vi "Client Read.vi"(7 "force configure? (F)":bool, 8 "error in":errorcluster, 11 "connection ID in":T1) -> (0 "error out":errorcluster, 3 "connection ID out":T1)   [LabVIEW 2010, in "NI_CCC.lvlib"]
doc: "Requests the latest values of the read tag list from the CCC server, and applies the values to the local CVT."
uses:
  NI_CCC.lvlib
  Connection ID.ctl
  <vilib>/NI/STM/TCP/TCP Connection Info.ctl
  <vilib>/NI/STM/SubVIs/MetaDataElement.ctl
  Tag Configuration.ctl
  <vilib>/NI/Current Value Table/Type Defs/Data Types.ctl
  Tag Direction.ctl
  <vilib>/NI/STM/TCP/TCP Read Options.ctl
  <vilib>/NI/STM/TCP/TCP Write Options.ctl
  <vilib>/NI/Current Value Table/Type Defs/Group Data.ctl
  <vilib>/NI/Current Value Table/Write grouped data to tags.vi
  Read Error.vi
  Initialize Address_Index Lists.vi
  <vilib>/NI/Current Value Table/Write Index Set.vi
  <vilib>/NI/Current Value Table/DataTypes/Double_Write Index Set.vi
  <vilib>/NI/Current Value Table/DataTypes/Array of String_Write Index Set.vi
  <vilib>/NI/Current Value Table/DataTypes/Array of Boolean_Write Index Set.vi
  <vilib>/NI/Current Value Table/DataTypes/Array of Single_Write Index Set.vi
  <vilib>/NI/Current Value Table/DataTypes/Array of Double_Write Index Set.vi
  <vilib>/NI/Current Value Table/DataTypes/Array of I8_Write Index Set.vi
  <vilib>/NI/Current Value Table/DataTypes/Array of I16_Write Index Set.vi
  <vilib>/NI/Current Value Table/DataTypes/Array of I32_Write Index Set.vi
  <vilib>/NI/Current Value Table/DataTypes/Array of I64_Write Index Set.vi
  <vilib>/NI/Current Value Table/DataTypes/Array of U64_Write Index Set.vi
  <vilib>/NI/Current Value Table/DataTypes/Array of U32_Write Index Set.vi
  <vilib>/NI/Current Value Table/DataTypes/Array of U16_Write Index Set.vi
  <vilib>/NI/Current Value Table/DataTypes/Array of U8_Write Index Set.vi
  <vilib>/NI/Current Value Table/DataTypes/Boolean_Write Index Set.vi
  <vilib>/NI/Current Value Table/DataTypes/String_Write Index Set.vi
  <vilib>/NI/Current Value Table/DataTypes/U8_Write Index Set.vi
  <vilib>/NI/Current Value Table/DataTypes/U16_Write Index Set.vi
  <vilib>/NI/Current Value Table/DataTypes/U32_Write Index Set.vi
  <vilib>/NI/Current Value Table/DataTypes/U64_Write Index Set.vi
  <vilib>/NI/Current Value Table/DataTypes/I8_Write Index Set.vi
  <vilib>/NI/Current Value Table/DataTypes/I16_Write Index Set.vi
  <vilib>/NI/Current Value Table/DataTypes/I32_Write Index Set.vi
  <vilib>/NI/Current Value Table/DataTypes/I64_Write Index Set.vi
  <vilib>/NI/Current Value Table/DataTypes/Single_Write Index Set.vi
  <vilib>/NI/Current Value Table/Get Index and Type.vi
  <vilib>/NI/Current Value Table/Group Tags.vi
  <vilib>/Utility/error.llb/Error Cluster From Error Code.vi
  FG Client Configurations.vi
  <vilib>/NI/Current Value Table/FGVs/Tag Memory.vi
  <vilib>/NI/Current Value Table/FGVs/Group Memory.vi
  <vilib>/NI/Current Value Table/Form Single Group.vi
  <vilib>/NI/Current Value Table/Memory Block.vi
  <vilib>/NI/Current Value Table/DataTypes/Double_Memory Block.vi
  <vilib>/NI/Current Value Table/DataTypes/Array of String_Memory Block.vi
  <vilib>/NI/Current Value Table/DataTypes/Array of Boolean_Memory Block.vi
  <vilib>/NI/Current Value Table/DataTypes/Array of Single_Memory Block.vi
  <vilib>/NI/Current Value Table/DataTypes/Array of Double_Memory Block.vi
  <vilib>/NI/Current Value Table/DataTypes/Array of I8_Memory Block.vi
  <vilib>/NI/Current Value Table/DataTypes/Array of I16_Memory Block.vi
  <vilib>/NI/Current Value Table/DataTypes/Array of I32_Memory Block.vi
  <vilib>/NI/Current Value Table/DataTypes/Array of I64_Memory Block.vi
  <vilib>/NI/Current Value Table/DataTypes/Array of U64_Memory Block.vi
  <vilib>/NI/Current Value Table/DataTypes/Array of U32_Memory Block.vi
  <vilib>/NI/Current Value Table/DataTypes/Array of U16_Memory Block.vi
  <vilib>/NI/Current Value Table/DataTypes/Array of U8_Memory Block.vi
  <vilib>/NI/Current Value Table/DataTypes/Boolean_Memory Block.vi
  <vilib>/NI/Current Value Table/DataTypes/String_Memory Block.vi
  <vilib>/NI/Current Value Table/DataTypes/U8_Memory Block.vi
  <vilib>/NI/Current Value Table/DataTypes/U16_Memory Block.vi
  <vilib>/NI/Current Value Table/DataTypes/U32_Memory Block.vi
  <vilib>/NI/Current Value Table/DataTypes/U64_Memory Block.vi
  <vilib>/NI/Current Value Table/DataTypes/I8_Memory Block.vi
  <vilib>/NI/Current Value Table/DataTypes/I16_Memory Block.vi
  <vilib>/NI/Current Value Table/DataTypes/I32_Memory Block.vi
  <vilib>/NI/Current Value Table/DataTypes/I64_Memory Block.vi
  <vilib>/NI/Current Value Table/DataTypes/Single_Memory Block.vi
  <vilib>/NI/STM/NI STM.lvlib
  <vilib>/NI/Current Value Table/Current Value Table.lvlib
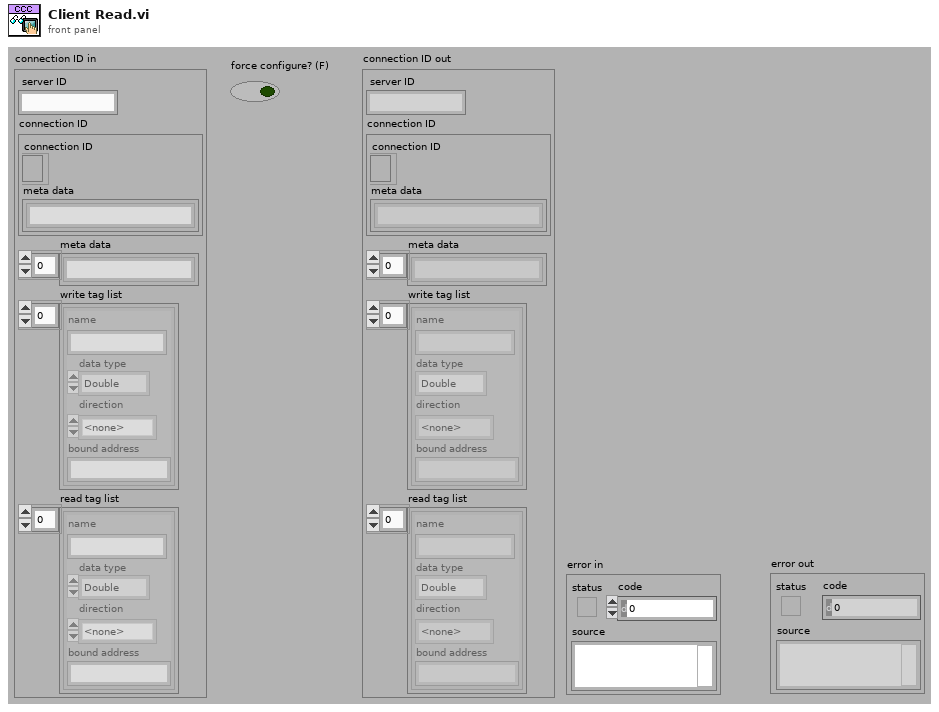
[diagram p1: front panel]
types:
  T1 = typedef "NI_CCC.lvlib/Connection ID.ctl" = cluster{"server ID":string, "connection ID":T2, "meta data":T3[], "write tag list":T4[], "read tag list":T4[]}
  T2 = typedef "NI STM.lvlib/TCP Connection Info.ctl" = cluster{"connection ID":refnum<k5>, "meta data":T3[]}
  T3 = typedef "NI STM.lvlib/MetaDataElement.ctl" = string
  T4 = typedef "NI_CCC.lvlib/Tag Configuration.ctl" = cluster{"name":string, "data type":T5, "direction":T6, "bound address":string}
  T5 = typedef "Current Value Table.lvlib/Data Types.ctl" = enum16{"Double", "Single", "I64", "I32", "I16", "I8", "U64", "U32", "U16", "U8", "String", "Boolean", "Array of U8", "Array of U16", "Array of U32", "Array of U64", "Array of I64", "Array of I32", "Array of I16", "Array of I8", "Array of Double", "Array of Single", "Array of Boolean", "Array of String"}
  T6 = typedef "NI_CCC.lvlib/Tag Direction.ctl" = enum32{"<none>", "Read", "Write"}
  T7 = typedef "NI STM.lvlib/TCP Read Options.ctl" = cluster{"ignore timeout error":bool, "timeout ms (1000)":i32}
  T8 = typedef "NI STM.lvlib/TCP Write Options.ctl" = cluster{"ignore timeout error":bool, "timeout ms (1000)":i32}
  T9 = typedef "Current Value Table.lvlib/Group Data.ctl" = cluster{"Double":dbl[], "Single":sgl[], "I64":i64[], "I32":i32[], "I16":i16[], "I8":i8[], "U64":u64[], "U32":u32[], "U16":u16[], "U8":u8[], "String":string[], "Boolean":bool[], "Array of U8":cluster{"U8 Array":u8[]}[], "Array of U16":cluster{"U16 Array":u16[]}[], "Array of U32":cluster{"U32 Array":u32[]}[], "Array of U64":cluster{"U64 Array":u64[]}[], "Array of I64":cluster{"I64 Array":i64[]}[], "Array of I32":cluster{"I32 Array":i32[]}[], "Array of I16":cluster{"I16 Array":i16[]}[], "Array of I8":cluster{"I8 Array":i8[]}[], "Array of Double":cluster{"DBL Array":dbl[]}[], "Array of Single":cluster{"SGL Array":sgl[]}[], "Array of Boolean":cluster{"Boolean Array":bool[]}[], "Array of String":cluster{"String Array":string[]}[]}
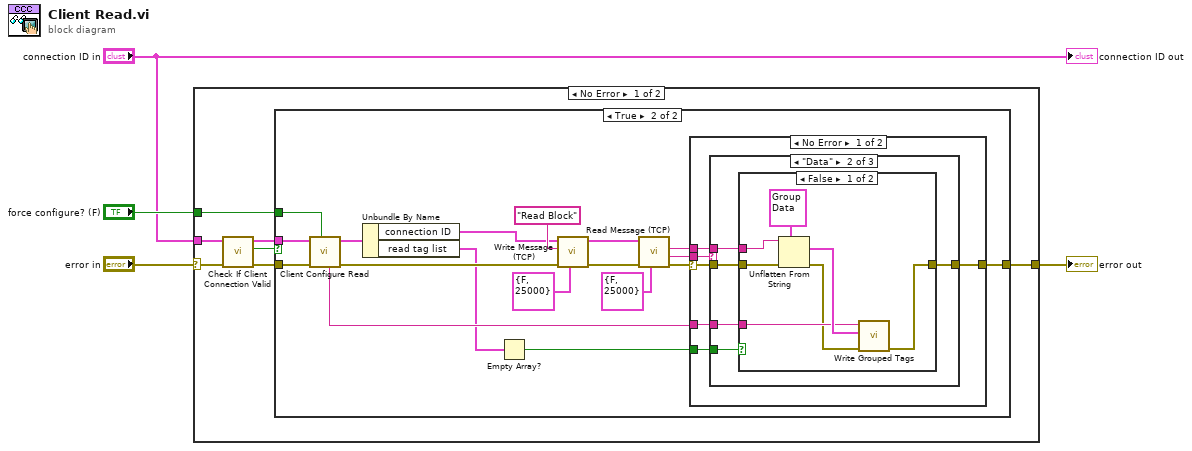
[diagram p0: block diagram]
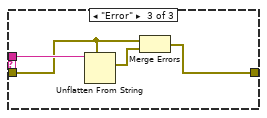
[diagram p5: hidden frame]
diagram:
  n1 = case shown="No Error" "error in" {
    selector: "error in" -> [w6 w56]
    tunnel: [w11 w56] -> w4
    tunnel: "force configure? (F)" -> [w10 _]
    tunnel: "connection ID in" -> [w9 _]
    frame No Error {
      n2 = call "Check If Client Connection Valid.vi"("error in"=w6, "connection ID in"=w9) -> ("error out"=w5:errorcluster, "valid?"=w8:bool, "connection ID out"=w7:T1)  [unwired: 7 in]
      n3 = case shown="True" w8 {
        tunnel: [w12 w24] -> w11
        tunnel: w5 -> [w12 w16]
        tunnel: w10 -> [_ w15]
        tunnel: w7 -> [_ w21]
        frame False {
        }
        frame True {
          n4 = call "Client Configure Read.vi"("force configure? (F)"=w15, "error in"=w16, "connection ID in"=w21) -> ("error out"=w17:errorcluster, "connection ID out"=w18:T1, "read group name"=w20:string)  [unwired: 5 in, 1 out]
          n5 = Unbundle By Name(w18) -> ("connection ID"=w19:T2, "read tag list"=w14:T4[])
          n6 = Empty Array?(array=w14) -> (empty?=w13:bool)
          n7 = call <vilib>:"Write Message (TCP).vi"("options"=T8 {"ignore timeout error"=FALSE, "timeout ms (1000)"=25000} ("Options"), "error in"=w17, "name"="Read Block" ("Name"), "connection info in"=w19) -> ("error out"=w27:errorcluster, "connection info out"=w26:T2)  [unwired: 6 in]
          n8 = call <vilib>:"Read Message (TCP).vi"("options"=T7 {"ignore timeout error"=FALSE, "timeout ms (1000)"=25000} ("Options"), "error in"=w27, "connection info in"=w26) -> ("error out"=w25:errorcluster, "name"=w29:T3, "data string"=w28:string)  [unwired: 3 in, 3 out]
          n9 = case shown="No Error" w25 {
            selector: w25 -> [w35 w55]
            tunnel: w29 -> [w32 _]
            tunnel: w28 -> [w36 _]
            tunnel: [w34 w55] -> w24
            tunnel: w20 -> [w33 _]
            tunnel: w13 -> [w31 _]
            frame No Error {
              n10 = case shown="\"Data\"" w32 {
                tunnel: w36 -> [_ w42 w53]
                tunnel: w35 -> [w37 w41 w52]
                tunnel: [w37 w39 w51] -> w34
                tunnel: w33 -> [_ w40 _]
                tunnel: w31 -> [_ w38 _]
                frame Default {
                  # "Unexpected Command"
                }
                frame "Data" {
                  n11 = case shown="False" w38 {
                    tunnel: w42 -> [w49 _]
                    tunnel: w41 -> [w48 w50]
                    tunnel: w40 -> [w45 _]
                    tunnel: [w43 w50] -> w39
                    frame False {
                      n12 = Unflatten From String(type=T9 {"Double"=[], "Single"=[], "I64"=[], "I32"=[], "I16"=[], "I8"=[], "U64"=[], "U32"=[], "U16"=[], "U8"=[], "String"=[], "Boolean"=[], "Array of U8"=[], "Array of U16"=[], "Array of U32"=[], "Array of U64"=[], "Array of I64"=[], "Array of I32"=[], "Array of I16"=[], "Array of I8"=[], "Array of Double"=[], "Array of Single"=[], "Array of Boolean"=[], "Array of String"=[]} ("Data"), binary string=w49, error in (no error)=w48) -> (value=w46:T9, error out=w44:errorcluster)  [unwired: 3 out]
                      n13 = call <vilib>:"Write Grouped Tags.vi"("error in (no error)"=w44, "Data"=w46, "Group"=w45) -> ("error out"=w43:errorcluster)  [unwired: 8 in]
                    }
                    frame True {
                      # "Don't attempt to write to group if read tag list is empty."
                    }
                  }
                }
                frame "Error" {
                  n14 = Unflatten From String(type=w52, binary string=w53) -> (value=w54:errorcluster)  [unwired: 1 in, 4 out]
                  n15 = Merge Errors(w52, w54) -> (w51:errorcluster)
                }
              }
            }
            frame Error {
            }
          }
        }
      }
    }
    frame Error {
    }
  }
  "error out" <- w4
  "connection ID out" <- "connection ID in"
